vi "TimeSpeedLength_Extractor.vi"(0 "TriggerS1":bool, 1 "Start_T1_prev":u32, 2 "Stop_T1_prev":u32, 5 "TriggerS1_prev-1":bool, 7 "Sensors_Distance [mm]":u32=101, 9 "TriggerS2_prev-1":bool, 11 "TriggerS2":bool, 12 "Start_T2_prev":u32) -> (3 "Length   [mm]":dbl, 4 "TriggerS1_prev0":bool, 6 "Start_T1":u32, 8 "Stop_T1":u32, 10 "Start_T2":u32, 14 "Speed [m/s]":dbl, 15 "TriggerS2_prev0":bool)   [LabVIEW 2020]
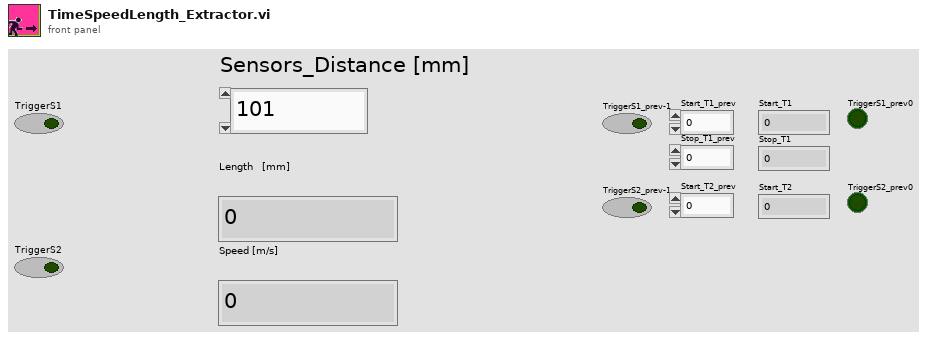
[diagram p1: front panel]
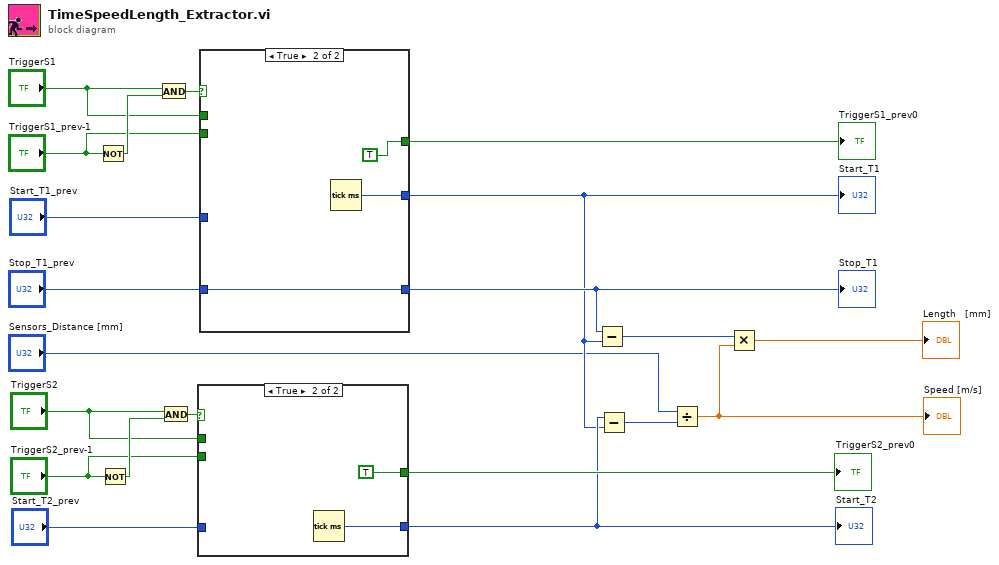
[diagram p0: block diagram]
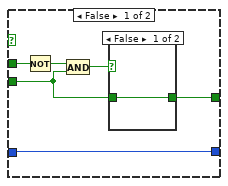
[diagram p2: hidden frame]
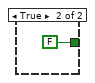
[diagram p3: hidden frame]
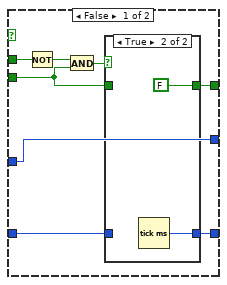
[diagram p4: hidden frame]
diagram:
  n1 = Not(x="TriggerS1_prev-1") -> (.not. x?=w21:bool)
  n2 = Not(x="TriggerS2_prev-1") -> (.not. x?=w14:bool)
  n3 = And(x="TriggerS1", y=w21) -> (x .and. y?=w20:bool)
  n4 = And(x="TriggerS2", y=w14) -> (x .and. y?=w13:bool)
  n5 = case shown="True" w13 {
    tunnel: "TriggerS2" -> [w27 _]
    tunnel: "TriggerS2_prev-1" -> [w23 _]
    tunnel: [w24 TRUE] -> w10
    tunnel: [w22 w30] -> w7
    tunnel: "Start_T2_prev" -> [w22 _]
    frame False {
      n6 = Not(x=w27) -> (.not. x?=w26:bool)
      n7 = And(x=w26, y=w23) -> (x .and. y?=w25:bool)
      n8 = case shown="False" w25 {
        tunnel: [w28 FALSE] -> w24
        tunnel: w23 -> [w28 _]
        frame False {
        }
        frame True {
        }
      }
    }
    frame True {
      n9 = Tick Count (ms)() -> (millisecond timer value=w30:u32)
    }
  }
  "TriggerS2_prev0" <- w10
  "Start_T2" <- w7
  n10 = case shown="True" w20 {
    tunnel: [w39 w46] -> w6
    tunnel: [w34 TRUE] -> w18
    tunnel: "Start_T1_prev" -> [w39 _]
    tunnel: "Stop_T1_prev" -> [w32 w44]
    tunnel: [w35 w44] -> w8
    tunnel: "TriggerS1" -> [w38 _]
    tunnel: "TriggerS1_prev-1" -> [w33 _]
    frame False {
      n11 = Not(x=w38) -> (.not. x?=w37:bool)
      n12 = And(x=w37, y=w33) -> (x .and. y?=w36:bool)
      n13 = case shown="True" w36 {
        tunnel: [w40 w43] -> w35
        tunnel: [w41 FALSE] -> w34
        tunnel: w33 -> [w41 _]
        tunnel: w32 -> [w40 _]
        frame False {
        }
        frame True {
          n14 = Tick Count (ms)() -> (millisecond timer value=w43:u32)
        }
      }
    }
    frame True {
      n15 = Tick Count (ms)() -> (millisecond timer value=w46:u32)
    }
  }
  "Start_T1" <- w6
  "TriggerS1_prev0" <- w18
  "Stop_T1" <- w8
  n16 = Subtract(x=w8, y=w6) -> (x-y=w3:u32)
  n17 = Subtract(x=w7, y=w6) -> (x-y=w5:u32)
  n18 = Divide(x="Sensors_Distance [mm]", y=w5) -> (x/y=w2:dbl)
  "Speed [m/s]" <- w2
  n19 = Multiply(x=w3, y=w2) -> (x*y=→"Length   [mm]":dbl)
